vi "CC Obervation Generate Telescope Focus Offset Step.vi"(8 "error in (no error)":errorcluster, 11 "Offset":dbl) -> (0 "error out":errorcluster, 3 "Steps":T1[](array[typedef]))   [LabVIEW 2024]
uses:
  typedefs/CC Script Step.ctl
  typedefs/CC enum Script Action.ctl
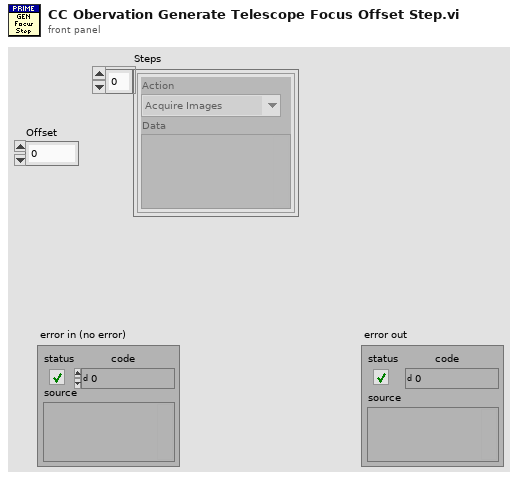
[diagram p1: front panel]
types:
  T1 = typedef "CC Script Step.ctl" = cluster{"Action":T2, "Data":variant}
  T2 = typedef "CC enum Script Action.ctl" = enum16{"Noop", "Define Object", "Define Exposure", "Define Dithering", "Acquire Images", "Set Filter Wheel", "Telescope Home", "Telescope Move", "Telescope RA DEC", "Focus Move Relative", "Focus Move Absolute", "Focus Set Home", "Macro", "Pause", "Ask User", "Define Random Dither"}
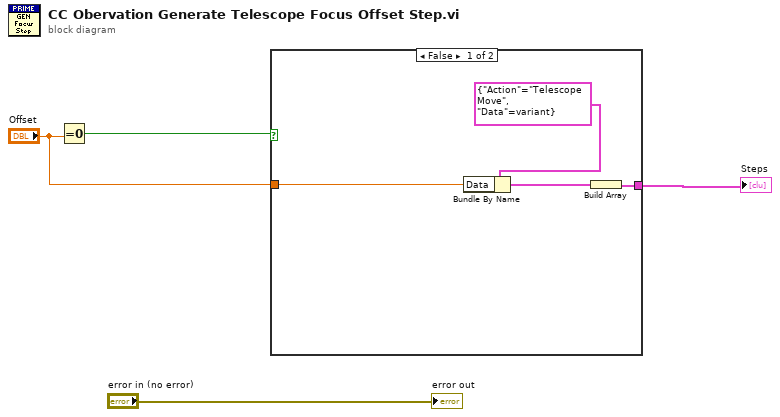
[diagram p0: block diagram]
diagram:
  n1 = Equal To 0?(x="Offset") -> (x = 0?=w3:bool)
  n2 = case shown="False" w3 {
    tunnel: [w5 _] -> w1
    tunnel: "Offset" -> [w6 _]
    frame False {
      n3 = Bundle By Name(cluster=T1 {"Action"=enum."Telescope Move", "Data"=variant}, "Data"=w6) -> (w7:T1)
      n4 = Build Array(w7) -> (w5:T1[])
    }
    frame True {
    }
  }
  "Steps" <- w1
  "error out" <- "error in (no error)"
